vi "Controller.vi"(0 "Path In":path, 1 "Inputs":cluster{"Numeric":dbl, "Boolean":bool}, 2 "Inputs 2":cluster{"Numeric":dbl, "Boolean":bool}, 3 "error in (no error)":errorcluster, 4 "Action":enum16{""}(ring), 6 "Settings":cluster{"Numeric":dbl, "Boolean":bool}) -> (7 "Path Out":path, 8 "Outputs":cluster{"Numeric":dbl, "Boolean":bool}, 9 "Outputs 2":cluster{"Numeric":dbl, "Boolean":bool}, 10 "error out":errorcluster)   [LabVIEW 2018]
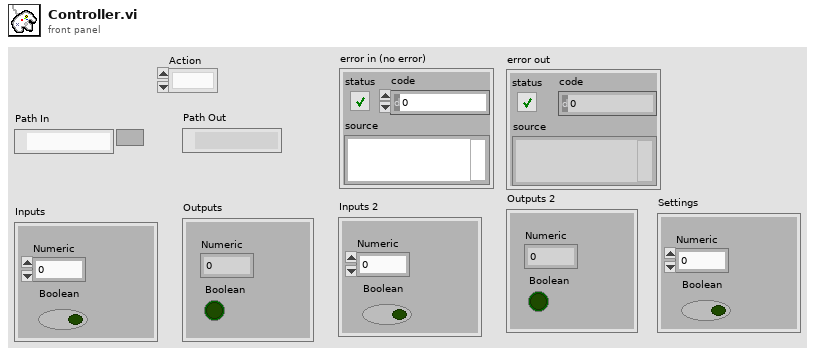
[diagram p1: front panel]
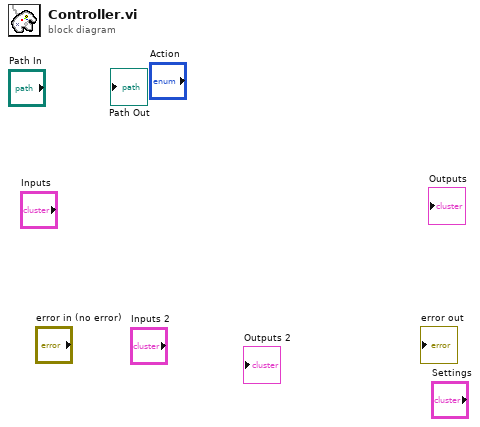
[diagram p0: block diagram]
diagram:
